vi "Read and Add Instr CFGs.vi"(8 "error in":errorcluster, 10 "Instr CFGs":path[](array[path]), 11 "File Provider in":refnum<class "File Provider.lvclass">) -> (0 "error out":errorcluster, 3 "File Provider out":refnum<class "File Provider.lvclass">)   [LabVIEW 2023, in "File Provider.lvlib" / "File Provider.lvclass"]
uses:
  File Provider.lvclass
  File Provider.lvclass/File Provider.ctl
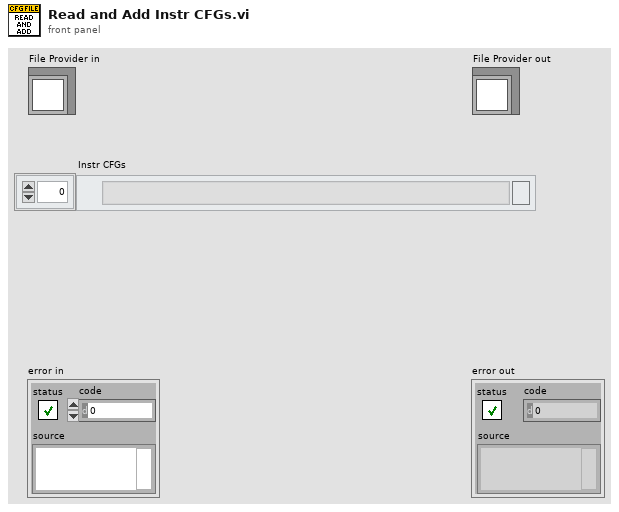
[diagram p1: front panel]
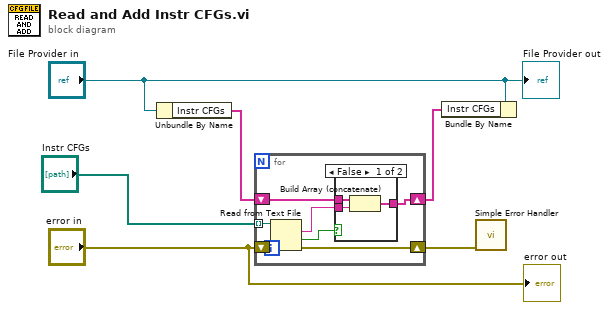
[diagram p0: block diagram]
diagram:
  n1 = Unbundle By Name("File Provider in") -> ("Instr CFGs"=w3:string[])
  n2 = for {
    tunnel: "Instr CFGs" -> [w8] mode=indexing
    shift-right: [w13] -> w6
    shift-left: "error in" -> [w12]
    shift-right: [w7] -> w1
    shift-left: w3 -> [w10]
    n3 = Read from Text File(file (use dialog)=w8, error in=w12) -> (text=w9:string, cancelled=w11:bool, error out=w13:errorcluster)  [unwired: 2 in, 1 out]
    n4 = case shown="False" w11 {
      tunnel: w10 -> [w16 w17]
      tunnel: w9 -> [w15 _]
      tunnel: [w14 w17] -> w7
      frame False {
        n5 = Build Array (concatenate)(w16, w15) -> (w14:string[])
      }
      frame True {
      }
    }
  }
  n6 = Bundle By Name(cluster="File Provider in", "Instr CFGs"=w1) -> ()  [unwired: 1 out]
  n7 = call <vilib>:"Simple Error Handler.vi"("error in (no error)"=w6) -> ()  [unwired: 4 in, 5 out]
  "error out" <- "error in"
  "File Provider out" <- "File Provider in"
